vi "Generate Actor ID.vi"() -> (2 "Actor ID":string)   [LabVIEW 2018, in "Monitored Actor.lvlib" / "Monitored Actor.lvclass"]
doc: "Generates a unique ID for each actor\n\nCopyright: Hill AFB\nAuthored By: Derek Trepanier"
uses:
  Monitored Actor.lvclass
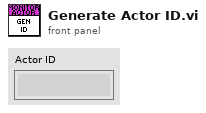
[diagram p1: front panel]
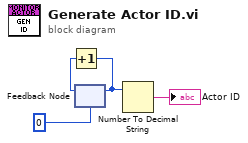
[diagram p0: block diagram]
diagram:
  n1 = feedback #1(0) -> (w3:i32)
  n2 = Increment(x=w3) -> (x+1=w2:i32)
  n3 = feedback-in #1(w2) -> ()
  n4 = Number To Decimal String(number=w2) -> (decimal integer string=→"Actor ID":string)  [unwired: 1 in]
